vi "Encoder Reset.vi"(9 "Use in Simulator (F)":bool, 11 "refnum name":string="My Encoder RefNum") -> ()   [LabVIEW 2012]
uses:
  Robot Global Data.vi
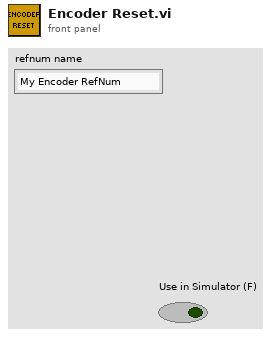
[diagram p1: front panel]
types:
  T1 = typedef "WPI_EncoderDevRef.ctl" = cluster{"DevStatus":errorcluster, "EncoderIndex":T2, "CounterIndex":T3, "DistancePerCount":dbl, "Decoding Type":T4}
  T2 = typedef "FPGA_EncoderIdx.ctl" = enum8{"Enc 0", "Enc 1", "Enc 2", "Enc 3", "Invalid"}
  T3 = typedef "FPGA_CounterCtrSystemIndex.ctl" = enum8{"Ctr 0", "Ctr 1", "Ctr 2", "Ctr 3", "Ctr 4", "Ctr 5", "Ctr 6", "Ctr 7", "Invalid"}
  T4 = typedef "WPI_EncoderType.ctl" = enum16{"1x", "2x", "4x"}
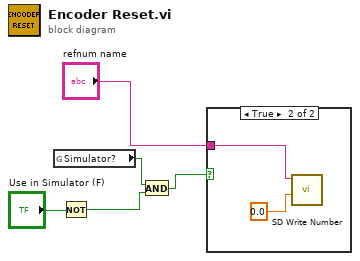
[diagram p0: block diagram]
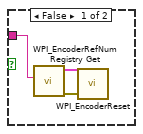
[diagram p2: hidden frame]
diagram:
  n1 = global read "Robot Global Data.vi" "Simulator?"() -> (w3:bool)
  n2 = Not(x="Use in Simulator (F)") -> (.not. x?=w2:bool)
  n3 = And(x=w3, y=w2) -> (x .and. y?=w1:bool)
  n4 = case shown="True" w1 {
    tunnel: "refnum name" -> [w6 w9]
    frame False {
      n5 = call <vilib>:"WPI_EncoderRefNum Registry Get.vi"("refnum name"=w6) -> ("error out"=w7:errorcluster, "EncoderDevRef"=w8:T1)  [unwired: 9 in]
      n6 = call <vilib>:"WPI_EncoderReset.vi"("error in (no error)"=w7, "EncoderDevRef"=w8) -> ()  [unwired: 8 in, 2 out]
    }
    frame True {
      n7 = call <vilib>:"SD Write Number.vi"("Numeric"=0.0, "Name"=w9) -> ()  [unwired: 8 in, 2 out]
    }
  }
